vi "Get Nested Tag Data.vi"(8 "error in (no error)":errorcluster, 10 "Path":cluster{"Tag ID / Name":variant, "Index":i32}[](array[cluster]), 11 "Raw Message in":refnum<class "Raw Message.lvclass">) -> (0 "error out":errorcluster, 1 "Tag Data":variant, 2 "Key not found?":bool, 3 "Raw Message out":refnum<class "Raw Message.lvclass">)   [LabVIEW 2020, in "Protobuf RAW.lvlib" / "Raw Message.lvclass"]
uses:
  Raw Message.lvclass
  Raw Message.lvclass/Raw Message.ctl
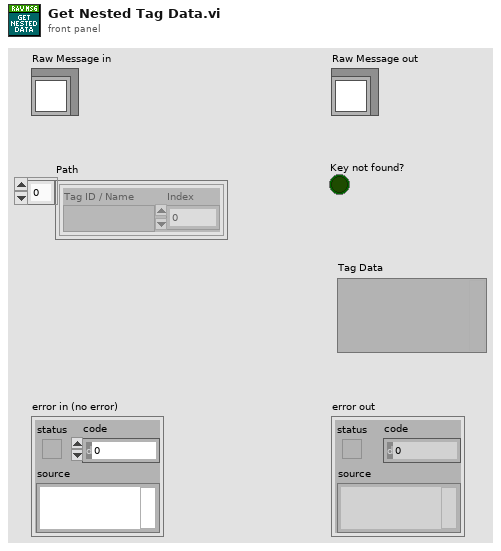
[diagram p1: front panel]
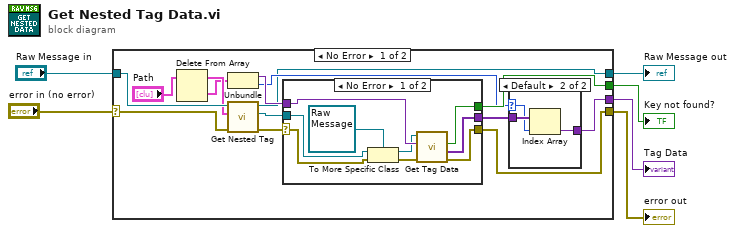
[diagram p0: block diagram]
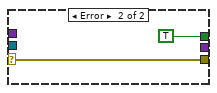
[diagram p3: hidden frame]
diagram:
  n1 = case shown="No Error" "error in (no error)" {
    selector: "error in (no error)" -> [w20 w37]
    tunnel: [w14 w37] -> w5
    tunnel: [w8 w36] -> w3
    tunnel: "Raw Message in" -> [w19 w36]
    tunnel: [w13 _] -> w2
    tunnel: [w11 _] -> w1
    frame No Error {
      n2 = Delete From Array(array="Path") -> (deleted portion=w17:cluster{"Tag ID / Name":variant, "Index":i32}, array with subset deleted=w18:cluster{"Tag ID / Name":variant, "Index":i32}[])  [unwired: 2 in]
      n3 = Unbundle(w17) -> ("Tag ID / Name"=w16:variant, "Index"=w10:i32)
      n4 = call "Get Nested Tag.vi"("error in (no error)"=w20, "Path"=w18, "Raw Message in"=w19) -> ("error out"=w15:errorcluster, "Tag"=w9:refnum<class "Basic Type.lvclass">, "Nested Message"=w8:refnum<class "Raw Message.lvclass">)  [unwired: 6 in]
      n5 = case shown="No Error" w15 {
        selector: w15 -> [w32 w34]
        tunnel: w16 -> [w33 _]
        tunnel: w9 -> [w27 _]
        tunnel: [w31 w34] -> w14
        tunnel: [w30 TRUE ("Key not found?")] -> w13
        tunnel: [w29 _] -> w12
        frame No Error {
          n6 = To More Specific Class(target class=refnum<class "Raw Message.lvclass"> refnum ("Protobuf RAW.lvlib:Raw Message.lvclass"), reference=w27, error in=w32) -> (specific class reference=w26:refnum<class "Raw Message.lvclass">, error out=w28:errorcluster)
          n7 = call "Get Tag Data.vi"("error in (no error)"=w28, "Tag ID"=w33, "Raw Message in"=w26) -> ("error out"=w31:errorcluster, "Tag Data"=w29:variant[], "Key not found?"=w30:bool)  [unwired: 5 in, 1 out]
        }
        frame Error {
        }
      }
      n8 = case shown="Default" w10 {
        selector: w10 -> [_ w22]
        tunnel: w12 -> [w21 w24]
        tunnel: [w21 w23] -> w11
        frame -1 {
        }
        frame Default {
          n9 = Index Array(array=w24, index=w22) -> (element=w23:variant)
        }
      }
    }
    frame Error {
    }
  }
  "error out" <- w5
  "Raw Message out" <- w3
  "Key not found?" <- w2
  "Tag Data" <- w1
